vi "JL_Obtain Temperature LED Config.vi"(0 "Temperature Option":u8 format="%x") -> (4 "Fail":bool, 6 "Pass":bool, 8 "Temperature LED Config":T1=enum."No Heat")   [LabVIEW 2016]
uses:
  type defs/Temp Setting Enum.ctl
panel:
  # "All integers are hex"
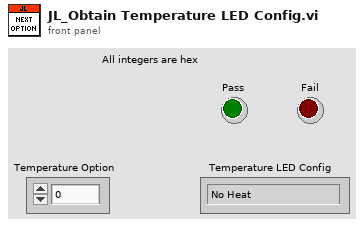
[diagram p1: front panel]
types:
  T1 = typedef "Temp Setting Enum.ctl" = enum16{"Off", "No Heat", "Extra Low", "Low", "Medium", "High", "*Incorrect*"}
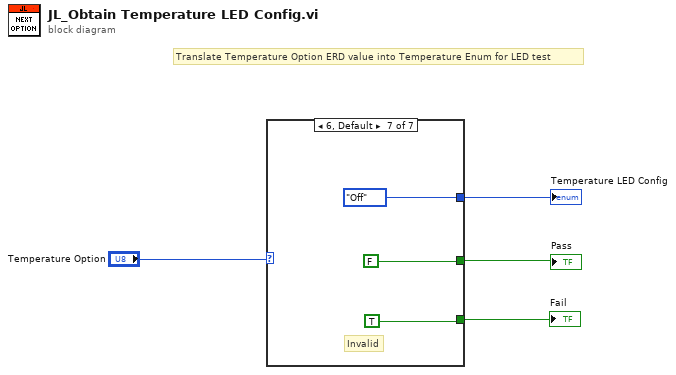
[diagram p0: block diagram]
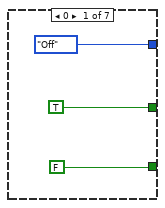
[diagram p2: hidden frame]
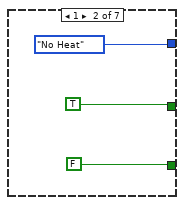
[diagram p3: hidden frame]
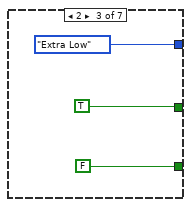
[diagram p4: hidden frame]
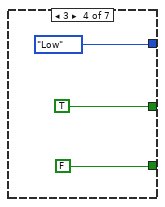
[diagram p5: hidden frame]
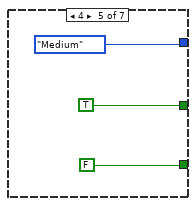
[diagram p6: hidden frame]
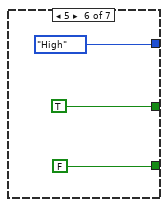
[diagram p7: hidden frame]
diagram:
  # "Translate Temperature Option ERD value into Temperature Enum for LED test"
  n1 = case shown="6, Default" "Temperature Option" {
    tunnel: [Temp_Setting_Enum."Off" ("Temp Setting 2") Temp_Setting_Enum."No Heat" ("Temp Setting 2") Temp_Setting_Enum."Extra Low" ("Temp Setting 2") Temp_Setting_Enum."Low" ("Temp Setting 2") Temp_Setting_Enum."Medium" ("Temp Setting 2") Temp_Setting_Enum."High" ("Temp Setting 2") Temp_Setting_Enum."Off" ("Temp Setting 2")] -> w4
    tunnel: [TRUE ("Pass 2") TRUE ("Pass 2") TRUE ("Pass 2") TRUE ("Pass 2") TRUE ("Pass 2") TRUE ("Pass 2") FALSE ("Pass 2")] -> w2
    tunnel: [FALSE ("Pass 2") FALSE ("Pass 2") FALSE ("Pass 2") FALSE ("Pass 2") FALSE ("Pass 2") FALSE ("Pass 2") TRUE ("Pass 2")] -> w1
    frame 0 {
    }
    frame 1 {
    }
    frame 2 {
    }
    frame 3 {
    }
    frame 4 {
    }
    frame 5 {
    }
    frame 6, Default {
      # "Invalid"
    }
  }
  "Temperature LED Config" <- w4
  "Pass" <- w2
  "Fail" <- w1
